vi "LabVIEW_MQTT_Toolkit_V2.vi"() -> ()   [LabVIEW 2021] (continued)
                n1873 = Close File(refnum=w4546, error in=w4544) -> (path=w4533:path)  [unwired: 1 out]
              }
              frame 16 {
                w4616 = T14 2 items=["User Home"=0, "User Desktop"=1, "User Documents"=2, "User Application Data"=3, "User Preferences"=4, "User Temporary"=5, "Public Documents"=6, "Public Application Data"=7, "Public Preferences"=8, "Public Cache"=13, "System Core Libraries"=9, "System Installed Libraries"=10, "Application Files"=11, "Boot Volume Root"=12] ("system directory type")
                n1874 = Decimate 1D Array(w4643) -> (w4641:dbl[])
                n1875 = Search and Replace String(replace all?=TRUE ("replace all? (F)"), input string=w4611, search string="/") -> (result string=w4632:string)  [unwired: 5 in, 3 out]
                n1876 = for {
                  tunnel: [w4665] -> w4640 mode=indexing
                  tunnel: w4642 -> [w4663] mode=indexing
                  tunnel: w4641 -> [w4662] mode=indexing
                  tunnel: [w4662] -> w4639 mode=indexing
                  tunnel: w4638 -> [w4657]
                  tunnel: w4637 -> [w4656]
                  tunnel: w4636 -> [w4655] mode=indexing
                  tunnel: w4635 -> [w4654]
                  tunnel: [w4648] -> w4634
                  n1877 = Join Numbers(hi=w4657, lo=w4656) -> ((hi.lo)=w4659:u32)
                  n1878 = To Double Precision Float(number=w4655) -> (double precision float=w4660:dbl)
                  n1879 = Number To Decimal String(number=w4663) -> (decimal integer string=w4664:string)  [unwired: 1 in]
                  n1880 = Number To Fractional String(number=w4662, precision (6)=i16 3 ("width (-)")) -> (F-format string=w4666:string)  [unwired: 2 in]
                  n1881 = Divide(x=w4660, y=w4654) -> (x/y=w4661:dbl)
                  n1882 = Build Array(w4664, w4666) -> (w4665:string[])
                  n1883 = To Unsigned Quad Integer(1:w4659) -> (0:w4658:u64)
                  n1884 = call "Unix Time to Timestamp.vi"("Fractional Second"=w4661, "Unix Time (s)"=w4658) -> ("Timestamp"=w4649:timestamp)  [unwired: 8 in, 1 out]
                  n1885 = Format Date/Time String(seconds (now)=w4649, UTC format=TRUE) -> (date/time string=w4650:string)  [unwired: 1 in]
                  n1886 = Scan From String(format string="%<%x %H:%M:%S%3u>T", input string=w4650) -> (output 1=w4651:timestamp)  [unwired: 3 in, 3 out]
                  n1887 = To Double Precision Float(number=w4651) -> (double precision float=w4648:dbl)
                }
                n1888 = Concatenate Strings(w4609, "TimeStamp;MeasureINC_Y(Deg)", "\n") -> (w4625:string)
                n1889 = Concatenate Strings(w4632, "_" ("string"), "S_E_T.csv") -> (w4633:string)
                n1890 = call <vilib>:"Get System Directory.vi"("system directory type"=w4616) -> ("system directory"=w4626:path)  [unwired: 10 in]
                n1891 = Build Path(base path=w4626, name or relative path="Logfile") -> (appended path=w4627:path)
                n1892 = call <vilib>:"Check if File or Folder Exists.vi"("path"=w4627) -> ("file or folder exists?"=w4628:bool, "dup path"=w4629:path)  [unwired: 8 in, 1 out]
                n1893 = case shown="False" w4628 {
                  tunnel: w4629 -> [w4646 w4647]
                  tunnel: [w4645 w4647] -> w4630
                  frame False {
                    n1894 = Create Folder(path (use dialog)=w4646) -> (created path=w4645:path)  [unwired: 2 in, 2 out]
                  }
                  frame True {
                  }
                }
                n1895 = Build Path(base path=w4630, name or relative path=w4633) -> (appended path=w4631:path)
                n1896 = Open/Create/Replace File(file path (use dialog)=w4631, operation (0:open)=T11."open or create") -> (refnum out=w4624:refnum<file>, error out=w4622:errorcluster)  [unwired: 4 in, 1 out]
                n1897 = Write to Text File(file (use dialog)=w4624, text=w4625, error in=w4622) -> (refnum out=w4623:refnum<file>, error out=w4621:errorcluster)  [unwired: 1 in, 1 out]
                n1898 = Close File(refnum=w4623, error in=w4621) -> (path=w4610:path)  [unwired: 1 out]
              }
              frame 17 {
                w4675 = T14 2 items=["User Home"=0, "User Desktop"=1, "User Documents"=2, "User Application Data"=3, "User Preferences"=4, "User Temporary"=5, "Public Documents"=6, "Public Application Data"=7, "Public Preferences"=8, "Public Cache"=13, "System Core Libraries"=9, "System Installed Libraries"=10, "Application Files"=11, "Boot Volume Root"=12] ("system directory type")
                n1899 = Decimate 1D Array(w4705) -> (w4701:dbl[], w4703:dbl[])
                n1900 = Search and Replace String(replace all?=TRUE ("replace all? (F)"), input string=w4670, search string="/") -> (result string=w4691:string)  [unwired: 5 in, 3 out]
                n1901 = for {
                  tunnel: [w4730] -> w4702 mode=indexing
                  tunnel: w4704 -> [w4728] mode=indexing
                  tunnel: w4701 -> [w4725] mode=indexing
                  tunnel: w4703 -> [w4724] mode=indexing
                  tunnel: [w4725] -> w4700 mode=indexing
                  tunnel: [w4724] -> w4699 mode=indexing
                  tunnel: w4698 -> [w4719]
                  tunnel: w4697 -> [w4718]
                  tunnel: w4696 -> [w4717] mode=indexing
                  tunnel: w4695 -> [w4716]
                  tunnel: [w4710] -> w4694
                  tunnel: [w4710] -> w4693
                  n1902 = Join Numbers(hi=w4719, lo=w4718) -> ((hi.lo)=w4721:u32)
                  n1903 = To Double Precision Float(number=w4717) -> (double precision float=w4722:dbl)
                  n1904 = Number To Decimal String(number=w4728) -> (decimal integer string=w4729:string)  [unwired: 1 in]
                  n1905 = Number To Fractional String(number=w4725, precision (6)=i16 3 ("width (-)")) -> (F-format string=w4731:string)  [unwired: 2 in]
                  n1906 = Number To Fractional String(number=w4724, precision (6)=i16 3 ("width (-)")) -> (F-format string=w4726:string)  [unwired: 2 in]
                  n1907 = Divide(x=w4722, y=w4716) -> (x/y=w4723:dbl)
                  n1908 = Build Array(w4729, w4731, w4726) -> (w4730:string[])
                  n1909 = To Unsigned Quad Integer(1:w4721) -> (0:w4720:u64)
                  n1910 = call "Unix Time to Timestamp.vi"("Fractional Second"=w4723, "Unix Time (s)"=w4720) -> ("Timestamp"=w4711:timestamp)  [unwired: 8 in, 1 out]
                  n1911 = Format Date/Time String(seconds (now)=w4711, UTC format=TRUE) -> (date/time string=w4712:string)  [unwired: 1 in]
                  n1912 = Scan From String(format string="%<%x %H:%M:%S%3u>T", input string=w4712) -> (output 1=w4713:timestamp)  [unwired: 3 in, 3 out]
                  n1913 = To Double Precision Float(number=w4713) -> (double precision float=w4710:dbl)
                }
                n1914 = Concatenate Strings(w4691, "_" ("string"), "S_E_T.csv") -> (w4692:string)
                n1915 = call <vilib>:"Get System Directory.vi"("system directory type"=w4675) -> ("system directory"=w4685:path)  [unwired: 10 in]
                n1916 = Concatenate Strings(w4668, "TimeStamp;MeasureCh_Z(g);INC_Y(Deg)", "\n") -> (w4684:string)
                n1917 = Build Path(base path=w4685, name or relative path="Logfile") -> (appended path=w4686:path)
                n1918 = call <vilib>:"Check if File or Folder Exists.vi"("path"=w4686) -> ("file or folder exists?"=w4687:bool, "dup path"=w4688:path)  [unwired: 8 in, 1 out]
                n1919 = case shown="False" w4687 {
                  tunnel: w4688 -> [w4708 w4709]
                  tunnel: [w4707 w4709] -> w4689
                  frame False {
                    n1920 = Create Folder(path (use dialog)=w4708) -> (created path=w4707:path)  [unwired: 2 in, 2 out]
                  }
                  frame True {
                  }
                }
                n1921 = Build Path(base path=w4689, name or relative path=w4692) -> (appended path=w4690:path)
                n1922 = Open/Create/Replace File(file path (use dialog)=w4690, operation (0:open)=T11."open or create") -> (refnum out=w4683:refnum<file>, error out=w4681:errorcluster)  [unwired: 4 in, 1 out]
                n1923 = Write to Text File(file (use dialog)=w4683, text=w4684, error in=w4681) -> (refnum out=w4682:refnum<file>, error out=w4680:errorcluster)  [unwired: 1 in, 1 out]
                n1924 = Close File(refnum=w4682, error in=w4680) -> (path=w4669:path)  [unwired: 1 out]
              }
              frame 18 {
                w4740 = T14 2 items=["User Home"=0, "User Desktop"=1, "User Documents"=2, "User Application Data"=3, "User Preferences"=4, "User Temporary"=5, "Public Documents"=6, "Public Application Data"=7, "Public Preferences"=8, "Public Cache"=13, "System Core Libraries"=9, "System Installed Libraries"=10, "Application Files"=11, "Boot Volume Root"=12] ("system directory type")
                n1925 = Decimate 1D Array(w4769) -> (w4765:dbl[], w4767:dbl[])
                n1926 = Search and Replace String(replace all?=TRUE ("replace all? (F)"), input string=w4734, search string="/") -> (result string=w4756:string)  [unwired: 5 in, 3 out]
                n1927 = Concatenate Strings(w4733, "TimeStamp;MeasureCh_X(g);INC_Y(Deg)", "\n") -> (w4749:string)
                n1928 = for {
                  tunnel: [w4794] -> w4766 mode=indexing
                  tunnel: w4768 -> [w4790] mode=indexing
                  tunnel: w4765 -> [w4789] mode=indexing
                  tunnel: w4767 -> [w4788] mode=indexing
                  tunnel: [w4789] -> w4764 mode=indexing
                  tunnel: [w4788] -> w4763 mode=indexing
                  tunnel: w4762 -> [w4783]
                  tunnel: w4761 -> [w4782]
                  tunnel: w4760 -> [w4781] mode=indexing
                  tunnel: w4759 -> [w4780]
                  tunnel: [w4774] -> w4758
                  n1929 = Join Numbers(hi=w4783, lo=w4782) -> ((hi.lo)=w4785:u32)
                  n1930 = To Double Precision Float(number=w4781) -> (double precision float=w4786:dbl)
                  n1931 = Number To Decimal String(number=w4790) -> (decimal integer string=w4793:string)  [unwired: 1 in]
                  n1932 = Number To Fractional String(number=w4789, precision (6)=i16 3 ("width (-)")) -> (F-format string=w4795:string)  [unwired: 2 in]
                  n1933 = Number To Fractional String(number=w4788, precision (6)=i16 3 ("width (-)")) -> (F-format string=w4791:string)  [unwired: 2 in]
                  n1934 = Divide(x=w4786, y=w4780) -> (x/y=w4787:dbl)
                  n1935 = Build Array(w4793, w4795, w4791) -> (w4794:string[])
                  n1936 = To Unsigned Quad Integer(1:w4785) -> (0:w4784:u64)
                  n1937 = call "Unix Time to Timestamp.vi"("Fractional Second"=w4787, "Unix Time (s)"=w4784) -> ("Timestamp"=w4775:timestamp)  [unwired: 8 in, 1 out]
                  n1938 = Format Date/Time String(seconds (now)=w4775, UTC format=TRUE) -> (date/time string=w4776:string)  [unwired: 1 in]
                  n1939 = Scan From String(format string="%<%x %H:%M:%S%3u>T", input string=w4776) -> (output 1=w4777:timestamp)  [unwired: 3 in, 3 out]
                  n1940 = To Double Precision Float(number=w4777) -> (double precision float=w4774:dbl)
                }
                n1941 = Concatenate Strings(w4756, "_" ("string"), "S_E_T.csv") -> (w4757:string)
                n1942 = call <vilib>:"Get System Directory.vi"("system directory type"=w4740) -> ("system directory"=w4750:path)  [unwired: 10 in]
                n1943 = Build Path(base path=w4750, name or relative path="Logfile") -> (appended path=w4751:path)
                n1944 = call <vilib>:"Check if File or Folder Exists.vi"("path"=w4751) -> ("file or folder exists?"=w4752:bool, "dup path"=w4753:path)  [unwired: 8 in, 1 out]
                n1945 = case shown="False" w4752 {
                  tunnel: w4753 -> [w4772 w4773]
                  tunnel: [w4771 w4773] -> w4754
                  frame False {
                    n1946 = Create Folder(path (use dialog)=w4772) -> (created path=w4771:path)  [unwired: 2 in, 2 out]
                  }
                  frame True {
                  }
                }
                n1947 = Build Path(base path=w4754, name or relative path=w4757) -> (appended path=w4755:path)
                n1948 = Open/Create/Replace File(file path (use dialog)=w4755, operation (0:open)=T11."open or create") -> (refnum out=w4748:refnum<file>, error out=w4746:errorcluster)  [unwired: 4 in, 1 out]
                n1949 = Write to Text File(file (use dialog)=w4748, text=w4749, error in=w4746) -> (refnum out=w4747:refnum<file>, error out=w4745:errorcluster)  [unwired: 1 in, 1 out]
                n1950 = Close File(refnum=w4747, error in=w4745) -> (path=w4735:path)  [unwired: 1 out]
              }
              frame 19 {
                w4804 = T14 2 items=["User Home"=0, "User Desktop"=1, "User Documents"=2, "User Application Data"=3, "User Preferences"=4, "User Temporary"=5, "Public Documents"=6, "Public Application Data"=7, "Public Preferences"=8, "Public Cache"=13, "System Core Libraries"=9, "System Installed Libraries"=10, "Application Files"=11, "Boot Volume Root"=12] ("system directory type")
                n1951 = Search and Replace String(replace all?=TRUE ("replace all? (F)"), input string=w4799, search string="/") -> (result string=w4820:string)  [unwired: 5 in, 3 out]
                n1952 = Concatenate Strings(w4820, "_" ("string"), "S_E_T.csv") -> (w4821:string)
                n1953 = call <vilib>:"Get System Directory.vi"("system directory type"=w4804) -> ("system directory"=w4814:path)  [unwired: 10 in]
                n1954 = Concatenate Strings(w4797, "TimeStamp;MeasureCh_Z(g);Ch_X(g);INC_Y(Deg)", "\n") -> (w4813:string)
                n1955 = Decimate 1D Array(w4837) -> (w4833:dbl[], w4832:dbl[], w4835:dbl[])
                n1956 = for {
                  tunnel: [w4865] -> w4834 mode=indexing
                  tunnel: w4836 -> [w4859] mode=indexing
                  tunnel: w4833 -> [w4858] mode=indexing
                  tunnel: w4832 -> [w4857] mode=indexing
                  tunnel: w4835 -> [w4856] mode=indexing
                  tunnel: [w4858] -> w4831 mode=indexing
                  tunnel: [w4857] -> w4830 mode=indexing
                  tunnel: [w4856] -> w4829 mode=indexing
                  tunnel: w4828 -> [w4851]
                  tunnel: w4827 -> [w4850]
                  tunnel: w4826 -> [w4849] mode=indexing
                  tunnel: w4825 -> [w4848]
                  tunnel: [w4842] -> w4824
                  tunnel: [w4842] -> w4823
                  tunnel: [w4842] -> w4822
                  n1957 = Join Numbers(hi=w4851, lo=w4850) -> ((hi.lo)=w4853:u32)
                  n1958 = To Double Precision Float(number=w4849) -> (double precision float=w4854:dbl)
                  n1959 = Number To Decimal String(number=w4859) -> (decimal integer string=w4864:string)  [unwired: 1 in]
                  n1960 = Number To Fractional String(number=w4858, precision (6)=i16 3 ("width (-)")) -> (F-format string=w4866:string)  [unwired: 2 in]
                  n1961 = Number To Fractional String(number=w4857, precision (6)=i16 3 ("width (-)")) -> (F-format string=w4862:string)  [unwired: 2 in]
                  n1962 = Number To Fractional String(number=w4856, precision (6)=i16 3 ("width (-)")) -> (F-format string=w4860:string)  [unwired: 2 in]
                  n1963 = Build Array(w4864, w4866, w4862, w4860) -> (w4865:string[])
                  n1964 = Divide(x=w4854, y=w4848) -> (x/y=w4855:dbl)
                  n1965 = To Unsigned Quad Integer(1:w4853) -> (0:w4852:u64)
                  n1966 = call "Unix Time to Timestamp.vi"("Fractional Second"=w4855, "Unix Time (s)"=w4852) -> ("Timestamp"=w4843:timestamp)  [unwired: 8 in, 1 out]
                  n1967 = Format Date/Time String(seconds (now)=w4843, UTC format=TRUE) -> (date/time string=w4844:string)  [unwired: 1 in]
                  n1968 = Scan From String(format string="%<%x %H:%M:%S%3u>T", input string=w4844) -> (output 1=w4845:timestamp)  [unwired: 3 in, 3 out]
                  n1969 = To Double Precision Float(number=w4845) -> (double precision float=w4842:dbl)
                }
                n1970 = Build Path(base path=w4814, name or relative path="Logfile") -> (appended path=w4815:path)
                n1971 = call <vilib>:"Check if File or Folder Exists.vi"("path"=w4815) -> ("file or folder exists?"=w4816:bool, "dup path"=w4817:path)  [unwired: 8 in, 1 out]
                n1972 = case shown="False" w4816 {
                  tunnel: w4817 -> [w4840 w4841]
                  tunnel: [w4839 w4841] -> w4818
                  frame False {
                    n1973 = Create Folder(path (use dialog)=w4840) -> (created path=w4839:path)  [unwired: 2 in, 2 out]
                  }
                  frame True {
                  }
                }
                n1974 = Build Path(base path=w4818, name or relative path=w4821) -> (appended path=w4819:path)
                n1975 = Open/Create/Replace File(file path (use dialog)=w4819, operation (0:open)=T11."open or create") -> (refnum out=w4812:refnum<file>, error out=w4810:errorcluster)  [unwired: 4 in, 1 out]
                n1976 = Write to Text File(file (use dialog)=w4812, text=w4813, error in=w4810) -> (refnum out=w4811:refnum<file>, error out=w4809:errorcluster)  [unwired: 1 in, 1 out]
                n1977 = Close File(refnum=w4811, error in=w4809) -> (path=w4798:path)  [unwired: 1 out]
              }
              frame 20 {
                w4875 = T14 2 items=["User Home"=0, "User Desktop"=1, "User Documents"=2, "User Application Data"=3, "User Preferences"=4, "User Temporary"=5, "Public Documents"=6, "Public Application Data"=7, "Public Preferences"=8, "Public Cache"=13, "System Core Libraries"=9, "System Installed Libraries"=10, "Application Files"=11, "Boot Volume Root"=12] ("system directory type")
                n1978 = Decimate 1D Array(w4904) -> (w4900:dbl[], w4902:dbl[])
                n1979 = Search and Replace String(replace all?=TRUE ("replace all? (F)"), input string=w4869, search string="/") -> (result string=w4891:string)  [unwired: 5 in, 3 out]
                n1980 = for {
                  tunnel: [w4929] -> w4901 mode=indexing
                  tunnel: w4903 -> [w4925] mode=indexing
                  tunnel: w4900 -> [w4924] mode=indexing
                  tunnel: w4902 -> [w4923] mode=indexing
                  tunnel: [w4924] -> w4899 mode=indexing
                  tunnel: [w4923] -> w4898 mode=indexing
                  tunnel: w4897 -> [w4918]
                  tunnel: w4896 -> [w4917]
                  tunnel: w4895 -> [w4916] mode=indexing
                  tunnel: w4894 -> [w4915]
                  tunnel: [w4909] -> w4893
                  n1981 = Join Numbers(hi=w4918, lo=w4917) -> ((hi.lo)=w4920:u32)
                  n1982 = To Double Precision Float(number=w4916) -> (double precision float=w4921:dbl)
                  n1983 = Number To Decimal String(number=w4925) -> (decimal integer string=w4928:string)  [unwired: 1 in]
                  n1984 = Number To Fractional String(number=w4924, precision (6)=i16 3 ("width (-)")) -> (F-format string=w4930:string)  [unwired: 2 in]
                  n1985 = Number To Fractional String(number=w4923, precision (6)=i16 3 ("width (-)")) -> (F-format string=w4926:string)  [unwired: 2 in]
                  n1986 = Divide(x=w4921, y=w4915) -> (x/y=w4922:dbl)
                  n1987 = Build Array(w4928, w4930, w4926) -> (w4929:string[])
                  n1988 = To Unsigned Quad Integer(1:w4920) -> (0:w4919:u64)
                  n1989 = call "Unix Time to Timestamp.vi"("Fractional Second"=w4922, "Unix Time (s)"=w4919) -> ("Timestamp"=w4910:timestamp)  [unwired: 8 in, 1 out]
                  n1990 = Format Date/Time String(seconds (now)=w4910, UTC format=TRUE) -> (date/time string=w4911:string)  [unwired: 1 in]
                  n1991 = Scan From String(format string="%<%x %H:%M:%S%3u>T", input string=w4911) -> (output 1=w4912:timestamp)  [unwired: 3 in, 3 out]
                  n1992 = To Double Precision Float(number=w4912) -> (double precision float=w4909:dbl)
                }
                n1993 = Concatenate Strings(w4868, "TimeStamp;MeasureCh_Y(g);INC_Y(Deg)", "\n") -> (w4884:string)
                n1994 = Concatenate Strings(w4891, "_" ("string"), "S_E_T.csv") -> (w4892:string)
                n1995 = call <vilib>:"Get System Directory.vi"("system directory type"=w4875) -> ("system directory"=w4885:path)  [unwired: 10 in]
                n1996 = Build Path(base path=w4885, name or relative path="Logfile") -> (appended path=w4886:path)
                n1997 = call <vilib>:"Check if File or Folder Exists.vi"("path"=w4886) -> ("file or folder exists?"=w4887:bool, "dup path"=w4888:path)  [unwired: 8 in, 1 out]
                n1998 = case shown="False" w4887 {
                  tunnel: w4888 -> [w4907 w4908]
                  tunnel: [w4906 w4908] -> w4889
                  frame False {
                    n1999 = Create Folder(path (use dialog)=w4907) -> (created path=w4906:path)  [unwired: 2 in, 2 out]
                  }
                  frame True {
                  }
                }
                n2000 = Build Path(base path=w4889, name or relative path=w4892) -> (appended path=w4890:path)
                n2001 = Open/Create/Replace File(file path (use dialog)=w4890, operation (0:open)=T11."open or create") -> (refnum out=w4883:refnum<file>, error out=w4881:errorcluster)  [unwired: 4 in, 1 out]
                n2002 = Write to Text File(file (use dialog)=w4883, text=w4884, error in=w4881) -> (refnum out=w4882:refnum<file>, error out=w4880:errorcluster)  [unwired: 1 in, 1 out]
                n2003 = Close File(refnum=w4882, error in=w4880) -> (path=w4870:path)  [unwired: 1 out]
              }
              frame 21 {
                w4939 = T14 2 items=["User Home"=0, "User Desktop"=1, "User Documents"=2, "User Application Data"=3, "User Preferences"=4, "User Temporary"=5, "Public Documents"=6, "Public Application Data"=7, "Public Preferences"=8, "Public Cache"=13, "System Core Libraries"=9, "System Installed Libraries"=10, "Application Files"=11, "Boot Volume Root"=12] ("system directory type")
                n2004 = Search and Replace String(replace all?=TRUE ("replace all? (F)"), input string=w4934, search string="/") -> (result string=w4955:string)  [unwired: 5 in, 3 out]
                n2005 = Concatenate Strings(w4932, "TimeStamp;MeasureCh_Z(g);Ch_Y(g);INC_Y(Deg)", "\n") -> (w4948:string)
                n2006 = Concatenate Strings(w4955, "_" ("string"), "S_E_T.csv") -> (w4956:string)
                n2007 = call <vilib>:"Get System Directory.vi"("system directory type"=w4939) -> ("system directory"=w4949:path)  [unwired: 10 in]
                n2008 = Decimate 1D Array(w4972) -> (w4968:dbl[], w4967:dbl[], w4970:dbl[])
                n2009 = for {
                  tunnel: [w5000] -> w4969 mode=indexing
                  tunnel: w4971 -> [w4994] mode=indexing
                  tunnel: w4968 -> [w4993] mode=indexing
                  tunnel: w4967 -> [w4992] mode=indexing
                  tunnel: w4970 -> [w4991] mode=indexing
                  tunnel: [w4993] -> w4966 mode=indexing
                  tunnel: [w4992] -> w4965 mode=indexing
                  tunnel: [w4991] -> w4964 mode=indexing
                  tunnel: w4963 -> [w4986]
                  tunnel: w4962 -> [w4985]
                  tunnel: w4961 -> [w4984] mode=indexing
                  tunnel: w4960 -> [w4983]
                  tunnel: [w4977] -> w4959
                  tunnel: [w4977] -> w4958
                  tunnel: [w4977] -> w4957
                  n2010 = Join Numbers(hi=w4986, lo=w4985) -> ((hi.lo)=w4988:u32)
                  n2011 = To Double Precision Float(number=w4984) -> (double precision float=w4989:dbl)
                  n2012 = Number To Decimal String(number=w4994) -> (decimal integer string=w4999:string)  [unwired: 1 in]
                  n2013 = Number To Fractional String(number=w4993, precision (6)=i16 3 ("width (-)")) -> (F-format string=w5001:string)  [unwired: 2 in]
                  n2014 = Number To Fractional String(number=w4992, precision (6)=i16 3 ("width (-)")) -> (F-format string=w4997:string)  [unwired: 2 in]
                  n2015 = Number To Fractional String(number=w4991, precision (6)=i16 3 ("width (-)")) -> (F-format string=w4995:string)  [unwired: 2 in]
                  n2016 = Build Array(w4999, w5001, w4997, w4995) -> (w5000:string[])
                  n2017 = Divide(x=w4989, y=w4983) -> (x/y=w4990:dbl)
                  n2018 = To Unsigned Quad Integer(1:w4988) -> (0:w4987:u64)
                  n2019 = call "Unix Time to Timestamp.vi"("Fractional Second"=w4990, "Unix Time (s)"=w4987) -> ("Timestamp"=w4978:timestamp)  [unwired: 8 in, 1 out]
                  n2020 = Format Date/Time String(seconds (now)=w4978, UTC format=TRUE) -> (date/time string=w4979:string)  [unwired: 1 in]
                  n2021 = Scan From String(format string="%<%x %H:%M:%S%3u>T", input string=w4979) -> (output 1=w4980:timestamp)  [unwired: 3 in, 3 out]
                  n2022 = To Double Precision Float(number=w4980) -> (double precision float=w4977:dbl)
                }
                n2023 = Build Path(base path=w4949, name or relative path="Logfile") -> (appended path=w4950:path)
                n2024 = call <vilib>:"Check if File or Folder Exists.vi"("path"=w4950) -> ("file or folder exists?"=w4951:bool, "dup path"=w4952:path)  [unwired: 8 in, 1 out]
                n2025 = case shown="False" w4951 {
                  tunnel: w4952 -> [w4975 w4976]
                  tunnel: [w4974 w4976] -> w4953
                  frame False {
                    n2026 = Create Folder(path (use dialog)=w4975) -> (created path=w4974:path)  [unwired: 2 in, 2 out]
                  }
                  frame True {
                  }
                }
                n2027 = Build Path(base path=w4953, name or relative path=w4956) -> (appended path=w4954:path)
                n2028 = Open/Create/Replace File(file path (use dialog)=w4954, operation (0:open)=T11."open or create") -> (refnum out=w4947:refnum<file>, error out=w4945:errorcluster)  [unwired: 4 in, 1 out]
                n2029 = Write to Text File(file (use dialog)=w4947, text=w4948, error in=w4945) -> (refnum out=w4946:refnum<file>, error out=w4944:errorcluster)  [unwired: 1 in, 1 out]
                n2030 = Close File(refnum=w4946, error in=w4944) -> (path=w4933:path)  [unwired: 1 out]
              }
              frame 22 {
                w5010 = T14 2 items=["User Home"=0, "User Desktop"=1, "User Documents"=2, "User Application Data"=3, "User Preferences"=4, "User Temporary"=5, "Public Documents"=6, "Public Application Data"=7, "Public Preferences"=8, "Public Cache"=13, "System Core Libraries"=9, "System Installed Libraries"=10, "Application Files"=11, "Boot Volume Root"=12] ("system directory type")
                n2031 = Search and Replace String(replace all?=TRUE ("replace all? (F)"), input string=w5005, search string="/") -> (result string=w5026:string)  [unwired: 5 in, 3 out]
                n2032 = Concatenate Strings(w5003, "TimeStamp;MeasureCh_X(g);Ch_Y(g);INC_X(Deg)", "\n") -> (w5019:string)
                n2033 = Concatenate Strings(w5026, "_" ("string"), "S_E_T.csv") -> (w5027:string)
                n2034 = call <vilib>:"Get System Directory.vi"("system directory type"=w5010) -> ("system directory"=w5020:path)  [unwired: 10 in]
                n2035 = Decimate 1D Array(w5043) -> (w5039:dbl[], w5038:dbl[], w5042:dbl[])
                n2036 = for {
                  tunnel: [w5071] -> w5040 mode=indexing
                  tunnel: w5041 -> [w5065] mode=indexing
                  tunnel: w5039 -> [w5064] mode=indexing
                  tunnel: w5038 -> [w5063] mode=indexing
                  tunnel: w5042 -> [w5062] mode=indexing
                  tunnel: [w5064] -> w5037 mode=indexing
                  tunnel: [w5063] -> w5036 mode=indexing
                  tunnel: [w5062] -> w5035 mode=indexing
                  tunnel: w5034 -> [w5057]
                  tunnel: w5033 -> [w5056]
                  tunnel: w5032 -> [w5055] mode=indexing
                  tunnel: w5031 -> [w5054]
                  tunnel: [w5048] -> w5030
                  tunnel: [w5048] -> w5029
                  tunnel: [w5048] -> w5028
                  n2037 = Join Numbers(hi=w5057, lo=w5056) -> ((hi.lo)=w5059:u32)
                  n2038 = To Double Precision Float(number=w5055) -> (double precision float=w5060:dbl)
                  n2039 = Number To Decimal String(number=w5065) -> (decimal integer string=w5070:string)  [unwired: 1 in]
                  n2040 = Number To Fractional String(number=w5064, precision (6)=i16 3 ("width (-)")) -> (F-format string=w5072:string)  [unwired: 2 in]
                  n2041 = Number To Fractional String(number=w5063, precision (6)=i16 3 ("width (-)")) -> (F-format string=w5068:string)  [unwired: 2 in]
                  n2042 = Number To Fractional String(number=w5062, precision (6)=i16 3 ("width (-)")) -> (F-format string=w5066:string)  [unwired: 2 in]
                  n2043 = Build Array(w5070, w5072, w5068, w5066) -> (w5071:string[])
                  n2044 = Divide(x=w5060, y=w5054) -> (x/y=w5061:dbl)
                  n2045 = To Unsigned Quad Integer(1:w5059) -> (0:w5058:u64)
                  n2046 = call "Unix Time to Timestamp.vi"("Fractional Second"=w5061, "Unix Time (s)"=w5058) -> ("Timestamp"=w5049:timestamp)  [unwired: 8 in, 1 out]
                  n2047 = Format Date/Time String(seconds (now)=w5049, UTC format=TRUE) -> (date/time string=w5050:string)  [unwired: 1 in]
                  n2048 = Scan From String(format string="%<%x %H:%M:%S%3u>T", input string=w5050) -> (output 1=w5051:timestamp)  [unwired: 3 in, 3 out]
                  n2049 = To Double Precision Float(number=w5051) -> (double precision float=w5048:dbl)
                }
                n2050 = Build Path(base path=w5020, name or relative path="Logfile") -> (appended path=w5021:path)
                n2051 = call <vilib>:"Check if File or Folder Exists.vi"("path"=w5021) -> ("file or folder exists?"=w5022:bool, "dup path"=w5023:path)  [unwired: 8 in, 1 out]
                n2052 = case shown="False" w5022 {
                  tunnel: w5023 -> [w5046 w5047]
                  tunnel: [w5045 w5047] -> w5024
                  frame False {
                    n2053 = Create Folder(path (use dialog)=w5046) -> (created path=w5045:path)  [unwired: 2 in, 2 out]
                  }
                  frame True {
                  }
                }
                n2054 = Build Path(base path=w5024, name or relative path=w5027) -> (appended path=w5025:path)
                n2055 = Open/Create/Replace File(file path (use dialog)=w5025, operation (0:open)=T11."open or create") -> (refnum out=w5018:refnum<file>, error out=w5016:errorcluster)  [unwired: 4 in, 1 out]
                n2056 = Write to Text File(file (use dialog)=w5018, text=w5019, error in=w5016) -> (refnum out=w5017:refnum<file>, error out=w5015:errorcluster)  [unwired: 1 in, 1 out]
                n2057 = Close File(refnum=w5017, error in=w5015) -> (path=w5004:path)  [unwired: 1 out]
              }
              frame 23 {
                w5081 = T14 2 items=["User Home"=0, "User Desktop"=1, "User Documents"=2, "User Application Data"=3, "User Preferences"=4, "User Temporary"=5, "Public Documents"=6, "Public Application Data"=7, "Public Preferences"=8, "Public Cache"=13, "System Core Libraries"=9, "System Installed Libraries"=10, "Application Files"=11, "Boot Volume Root"=12] ("system directory type")
                n2058 = Search and Replace String(replace all?=TRUE ("replace all? (F)"), input string=w5075, search string="/") -> (result string=w5097:string)  [unwired: 5 in, 3 out]
                n2059 = Concatenate Strings(w5074, "TimeStamp;MeasureCh_Z(g);Ch_X(g);Ch_Y(g);INC_Y(Deg)", "\n") -> (w5090:string)
                n2060 = Concatenate Strings(w5097, "_" ("string"), "S_E_T.csv") -> (w5098:string)
                n2061 = call <vilib>:"Get System Directory.vi"("system directory type"=w5081) -> ("system directory"=w5091:path)  [unwired: 10 in]
                n2062 = Decimate 1D Array(w5114) -> (w5113:dbl[], w5112:dbl[], w5111:dbl[], w5108:dbl[])
                n2063 = for {
                  tunnel: [w5144] -> w5109 mode=indexing
                  tunnel: w5110 -> [w5138] mode=indexing
                  tunnel: w5113 -> [w5136] mode=indexing
                  tunnel: w5112 -> [w5135] mode=indexing
                  tunnel: w5111 -> [w5134] mode=indexing
                  tunnel: w5108 -> [w5133] mode=indexing
                  tunnel: [w5136] -> w5107 mode=indexing
                  tunnel: [w5135] -> w5106 mode=indexing
                  tunnel: [w5134] -> w5105 mode=indexing
                  tunnel: [w5133] -> w5104 mode=indexing
                  tunnel: w5103 -> [w5128]
                  tunnel: w5102 -> [w5127]
                  tunnel: w5101 -> [w5126] mode=indexing
                  tunnel: w5100 -> [w5125]
                  tunnel: [w5119] -> w5099
                  n2064 = Number To Fractional String(number=w5133, precision (6)=i16 3 ("width (-)")) -> ()  [unwired: 2 in, 1 out]
                  n2065 = Join Numbers(hi=w5128, lo=w5127) -> ((hi.lo)=w5130:u32)
                  n2066 = To Double Precision Float(number=w5126) -> (double precision float=w5131:dbl)
                  n2067 = Number To Decimal String(number=w5138) -> (decimal integer string=w5143:string)  [unwired: 1 in]
                  n2068 = Number To Fractional String(number=w5136, precision (6)=i16 3 ("width (-)")) -> (F-format string=w5145:string)  [unwired: 2 in]
                  n2069 = Number To Fractional String(number=w5135, precision (6)=i16 3 ("width (-)")) -> (F-format string=w5141:string)  [unwired: 2 in]
                  n2070 = Number To Fractional String(number=w5134, precision (6)=i16 3 ("width (-)")) -> (F-format string=w5139:string)  [unwired: 2 in]
                  n2071 = Build Array(w5143, w5145, w5141, w5139) -> (w5144:string[])
                  n2072 = Divide(x=w5131, y=w5125) -> (x/y=w5132:dbl)
                  n2073 = To Unsigned Quad Integer(1:w5130) -> (0:w5129:u64)
                  n2074 = call "Unix Time to Timestamp.vi"("Fractional Second"=w5132, "Unix Time (s)"=w5129) -> ("Timestamp"=w5120:timestamp)  [unwired: 8 in, 1 out]
                  n2075 = Format Date/Time String(seconds (now)=w5120, UTC format=TRUE) -> (date/time string=w5121:string)  [unwired: 1 in]
                  n2076 = Scan From String(format string="%<%x %H:%M:%S%3u>T", input string=w5121) -> (output 1=w5122:timestamp)  [unwired: 3 in, 3 out]
                  n2077 = To Double Precision Float(number=w5122) -> (double precision float=w5119:dbl)
                }
                n2078 = Build Path(base path=w5091, name or relative path="Logfile") -> (appended path=w5092:path)
                n2079 = call <vilib>:"Check if File or Folder Exists.vi"("path"=w5092) -> ("file or folder exists?"=w5093:bool, "dup path"=w5094:path)  [unwired: 8 in, 1 out]
                n2080 = case shown="False" w5093 {
                  tunnel: w5094 -> [w5117 w5118]
                  tunnel: [w5116 w5118] -> w5095
                  frame False {
                    n2081 = Create Folder(path (use dialog)=w5117) -> (created path=w5116:path)  [unwired: 2 in, 2 out]
                  }
                  frame True {
                  }
                }
                n2082 = Build Path(base path=w5095, name or relative path=w5098) -> (appended path=w5096:path)
                n2083 = Open/Create/Replace File(file path (use dialog)=w5096, operation (0:open)=T11."open or create") -> (refnum out=w5089:refnum<file>, error out=w5087:errorcluster)  [unwired: 4 in, 1 out]
                n2084 = Write to Text File(file (use dialog)=w5089, text=w5090, error in=w5087) -> (refnum out=w5088:refnum<file>, error out=w5086:errorcluster)  [unwired: 1 in, 1 out]
                n2085 = Close File(refnum=w5088, error in=w5086) -> (path=w5076:path)  [unwired: 1 out]
              }
              frame 24 {
                w5154 = T14 2 items=["User Home"=0, "User Desktop"=1, "User Documents"=2, "User Application Data"=3, "User Preferences"=4, "User Temporary"=5, "Public Documents"=6, "Public Application Data"=7, "Public Preferences"=8, "Public Cache"=13, "System Core Libraries"=9, "System Installed Libraries"=10, "Application Files"=11, "Boot Volume Root"=12] ("system directory type")
                n2086 = Decimate 1D Array(w5183) -> (w5181:dbl[], w5180:dbl[])
                n2087 = Search and Replace String(replace all?=TRUE ("replace all? (F)"), input string=w5149, search string="/") -> (result string=w5170:string)  [unwired: 5 in, 3 out]
                n2088 = Concatenate Strings(w5147, "TimeStamp;Measure INC_X(Deg);INC_Y(Deg)", "\n") -> (w5163:string)
                n2089 = for {
                  tunnel: [w5208] -> w5179 mode=indexing
                  tunnel: w5182 -> [w5204] mode=indexing
                  tunnel: w5181 -> [w5203] mode=indexing
                  tunnel: w5180 -> [w5202] mode=indexing
                  tunnel: [w5203] -> w5178 mode=indexing
                  tunnel: [w5202] -> w5177 mode=indexing
                  tunnel: w5176 -> [w5197]
                  tunnel: w5175 -> [w5196]
                  tunnel: w5174 -> [w5195] mode=indexing
                  tunnel: w5173 -> [w5194]
                  tunnel: [w5188] -> w5172
                  n2090 = Join Numbers(hi=w5197, lo=w5196) -> ((hi.lo)=w5199:u32)
                  n2091 = To Double Precision Float(number=w5195) -> (double precision float=w5200:dbl)
                  n2092 = Number To Decimal String(number=w5204) -> (decimal integer string=w5207:string)  [unwired: 1 in]
                  n2093 = Number To Fractional String(number=w5203, precision (6)=i16 3 ("width (-)")) -> (F-format string=w5209:string)  [unwired: 2 in]
                  n2094 = Number To Fractional String(number=w5202, precision (6)=i16 3 ("width (-)")) -> (F-format string=w5205:string)  [unwired: 2 in]
                  n2095 = Divide(x=w5200, y=w5194) -> (x/y=w5201:dbl)
                  n2096 = Build Array(w5207, w5209, w5205) -> (w5208:string[])
                  n2097 = To Unsigned Quad Integer(1:w5199) -> (0:w5198:u64)
                  n2098 = call "Unix Time to Timestamp.vi"("Fractional Second"=w5201, "Unix Time (s)"=w5198) -> ("Timestamp"=w5189:timestamp)  [unwired: 8 in, 1 out]
                  n2099 = Format Date/Time String(seconds (now)=w5189, UTC format=TRUE) -> (date/time string=w5190:string)  [unwired: 1 in]
                  n2100 = Scan From String(format string="%<%x %H:%M:%S%3u>T", input string=w5190) -> (output 1=w5191:timestamp)  [unwired: 3 in, 3 out]
                  n2101 = To Double Precision Float(number=w5191) -> (double precision float=w5188:dbl)
                }
                n2102 = Concatenate Strings(w5170, "_" ("string"), "S_E_T.csv") -> (w5171:string)
                n2103 = call <vilib>:"Get System Directory.vi"("system directory type"=w5154) -> ("system directory"=w5164:path)  [unwired: 10 in]
                n2104 = Build Path(base path=w5164, name or relative path="Logfile") -> (appended path=w5165:path)
                n2105 = call <vilib>:"Check if File or Folder Exists.vi"("path"=w5165) -> ("file or folder exists?"=w5166:bool, "dup path"=w5167:path)  [unwired: 8 in, 1 out]
                n2106 = case shown="False" w5166 {
                  tunnel: w5167 -> [w5186 w5187]
                  tunnel: [w5185 w5187] -> w5168
                  frame False {
                    n2107 = Create Folder(path (use dialog)=w5186) -> (created path=w5185:path)  [unwired: 2 in, 2 out]
                  }
                  frame True {
                  }
                }
                n2108 = Build Path(base path=w5168, name or relative path=w5171) -> (appended path=w5169:path)
                n2109 = Open/Create/Replace File(file path (use dialog)=w5169, operation (0:open)=T11."open or create") -> (refnum out=w5162:refnum<file>, error out=w5160:errorcluster)  [unwired: 4 in, 1 out]
                n2110 = Write to Text File(file (use dialog)=w5162, text=w5163, error in=w5160) -> (refnum out=w5161:refnum<file>, error out=w5159:errorcluster)  [unwired: 1 in, 1 out]
                n2111 = Close File(refnum=w5161, error in=w5159) -> (path=w5148:path)  [unwired: 1 out]
              }
              frame 25 {
                w5218 = T14 2 items=["User Home"=0, "User Desktop"=1, "User Documents"=2, "User Application Data"=3, "User Preferences"=4, "User Temporary"=5, "Public Documents"=6, "Public Application Data"=7, "Public Preferences"=8, "Public Cache"=13, "System Core Libraries"=9, "System Installed Libraries"=10, "Application Files"=11, "Boot Volume Root"=12] ("system directory type")
                n2112 = Search and Replace String(replace all?=TRUE ("replace all? (F)"), input string=w5213, search string="/") -> (result string=w5234:string)  [unwired: 5 in, 3 out]
                n2113 = Concatenate Strings(w5211, "TimeStamp;Measure Ch_Z(g);INC_X(Deg);INC_Y(Deg)", "\n") -> (w5227:string)
                n2114 = Concatenate Strings(w5234, "_" ("string"), "S_E_T.csv") -> (w5235:string)
                n2115 = call <vilib>:"Get System Directory.vi"("system directory type"=w5218) -> ("system directory"=w5228:path)  [unwired: 10 in]
                n2116 = Decimate 1D Array(w5249) -> (w5244:dbl[], w5247:dbl[], w5246:dbl[])
                n2117 = for {
                  tunnel: [w5277] -> w5245 mode=indexing
                  tunnel: w5248 -> [w5271] mode=indexing
                  tunnel: w5244 -> [w5270] mode=indexing
                  tunnel: w5247 -> [w5269] mode=indexing
                  tunnel: w5246 -> [w5268] mode=indexing
                  tunnel: [w5270] -> w5243 mode=indexing
                  tunnel: [w5269] -> w5242 mode=indexing
                  tunnel: [w5268] -> w5241 mode=indexing
                  tunnel: w5240 -> [w5263]
                  tunnel: w5239 -> [w5262]
                  tunnel: w5238 -> [w5261] mode=indexing
                  tunnel: w5237 -> [w5260]
                  tunnel: [w5254] -> w5236
                  n2118 = Join Numbers(hi=w5263, lo=w5262) -> ((hi.lo)=w5265:u32)
                  n2119 = To Double Precision Float(number=w5261) -> (double precision float=w5266:dbl)
                  n2120 = Number To Decimal String(number=w5271) -> (decimal integer string=w5276:string)  [unwired: 1 in]
                  n2121 = Number To Fractional String(number=w5270, precision (6)=i16 3 ("width (-)")) -> (F-format string=w5278:string)  [unwired: 2 in]
                  n2122 = Number To Fractional String(number=w5269, precision (6)=i16 3 ("width (-)")) -> (F-format string=w5274:string)  [unwired: 2 in]
                  n2123 = Number To Fractional String(number=w5268, precision (6)=i16 3 ("width (-)")) -> (F-format string=w5272:string)  [unwired: 2 in]
                  n2124 = Build Array(w5276, w5278, w5274, w5272) -> (w5277:string[])
                  n2125 = Divide(x=w5266, y=w5260) -> (x/y=w5267:dbl)
                  n2126 = To Unsigned Quad Integer(1:w5265) -> (0:w5264:u64)
                  n2127 = call "Unix Time to Timestamp.vi"("Fractional Second"=w5267, "Unix Time (s)"=w5264) -> ("Timestamp"=w5255:timestamp)  [unwired: 8 in, 1 out]
                  n2128 = Format Date/Time String(seconds (now)=w5255, UTC format=TRUE) -> (date/time string=w5256:string)  [unwired: 1 in]
                  n2129 = Scan From String(format string="%<%x %H:%M:%S%3u>T", input string=w5256) -> (output 1=w5257:timestamp)  [unwired: 3 in, 3 out]
                  n2130 = To Double Precision Float(number=w5257) -> (double precision float=w5254:dbl)
                }
                n2131 = Build Path(base path=w5228, name or relative path="Logfile") -> (appended path=w5229:path)
                n2132 = call <vilib>:"Check if File or Folder Exists.vi"("path"=w5229) -> ("file or folder exists?"=w5230:bool, "dup path"=w5231:path)  [unwired: 8 in, 1 out]
                n2133 = case shown="False" w5230 {
                  tunnel: w5231 -> [w5252 w5253]
                  tunnel: [w5251 w5253] -> w5232
                  frame False {
                    n2134 = Create Folder(path (use dialog)=w5252) -> (created path=w5251:path)  [unwired: 2 in, 2 out]
                  }
                  frame True {
                  }
                }
                n2135 = Build Path(base path=w5232, name or relative path=w5235) -> (appended path=w5233:path)
                n2136 = Open/Create/Replace File(file path (use dialog)=w5233, operation (0:open)=T11."open or create") -> (refnum out=w5226:refnum<file>, error out=w5224:errorcluster)  [unwired: 4 in, 1 out]
                n2137 = Write to Text File(file (use dialog)=w5226, text=w5227, error in=w5224) -> (refnum out=w5225:refnum<file>, error out=w5223:errorcluster)  [unwired: 1 in, 1 out]
                n2138 = Close File(refnum=w5225, error in=w5223) -> (path=w5212:path)  [unwired: 1 out]
              }
              frame 26 {
                w5287 = T14 2 items=["User Home"=0, "User Desktop"=1, "User Documents"=2, "User Application Data"=3, "User Preferences"=4, "User Temporary"=5, "Public Documents"=6, "Public Application Data"=7, "Public Preferences"=8, "Public Cache"=13, "System Core Libraries"=9, "System Installed Libraries"=10, "Application Files"=11, "Boot Volume Root"=12] ("system directory type")
                n2139 = Search and Replace String(replace all?=TRUE ("replace all? (F)"), input string=w5282, search string="/") -> (result string=w5303:string)  [unwired: 5 in, 3 out]
                n2140 = Concatenate Strings(w5280, "TimeStamp;Measure Ch_X(g);INC_X(Deg);INC_Y(Deg)", "\n") -> (w5296:string)
                n2141 = Concatenate Strings(w5303, "_" ("string"), "S_E_T.csv") -> (w5304:string)
                n2142 = call <vilib>:"Get System Directory.vi"("system directory type"=w5287) -> ("system directory"=w5297:path)  [unwired: 10 in]
                n2143 = Decimate 1D Array(w5318) -> (w5313:dbl[], w5317:dbl[], w5316:dbl[])
                n2144 = for {
                  tunnel: [w5346] -> w5314 mode=indexing
                  tunnel: w5315 -> [w5340] mode=indexing
                  tunnel: w5313 -> [w5339] mode=indexing
                  tunnel: w5317 -> [w5338] mode=indexing
                  tunnel: w5316 -> [w5337] mode=indexing
                  tunnel: [w5339] -> w5312 mode=indexing
                  tunnel: [w5338] -> w5311 mode=indexing
                  tunnel: [w5337] -> w5310 mode=indexing
                  tunnel: w5309 -> [w5332]
                  tunnel: w5308 -> [w5331]
                  tunnel: w5307 -> [w5330] mode=indexing
                  tunnel: w5306 -> [w5329]
                  tunnel: [w5323] -> w5305
                  n2145 = Join Numbers(hi=w5332, lo=w5331) -> ((hi.lo)=w5334:u32)
                  n2146 = To Double Precision Float(number=w5330) -> (double precision float=w5335:dbl)
                  n2147 = Number To Decimal String(number=w5340) -> (decimal integer string=w5345:string)  [unwired: 1 in]
                  n2148 = Number To Fractional String(number=w5339, precision (6)=i16 3 ("width (-)")) -> (F-format string=w5347:string)  [unwired: 2 in]
                  n2149 = Number To Fractional String(number=w5338, precision (6)=i16 3 ("width (-)")) -> (F-format string=w5343:string)  [unwired: 2 in]
                  n2150 = Number To Fractional String(number=w5337, precision (6)=i16 3 ("width (-)")) -> (F-format string=w5341:string)  [unwired: 2 in]
                  n2151 = Build Array(w5345, w5347, w5343, w5341) -> (w5346:string[])
                  n2152 = Divide(x=w5335, y=w5329) -> (x/y=w5336:dbl)
                  n2153 = To Unsigned Quad Integer(1:w5334) -> (0:w5333:u64)
                  n2154 = call "Unix Time to Timestamp.vi"("Fractional Second"=w5336, "Unix Time (s)"=w5333) -> ("Timestamp"=w5324:timestamp)  [unwired: 8 in, 1 out]
                  n2155 = Format Date/Time String(seconds (now)=w5324, UTC format=TRUE) -> (date/time string=w5328:string)  [unwired: 1 in]
                  n2156 = Scan From String(format string="%<%x %H:%M:%S%3u>T", input string=w5328) -> (output 1=w5327:timestamp)  [unwired: 3 in, 3 out]
                  n2157 = To Double Precision Float(number=w5327) -> (double precision float=w5323:dbl)
                }
                n2158 = Build Path(base path=w5297, name or relative path="Logfile") -> (appended path=w5298:path)
                n2159 = call <vilib>:"Check if File or Folder Exists.vi"("path"=w5298) -> ("file or folder exists?"=w5299:bool, "dup path"=w5300:path)  [unwired: 8 in, 1 out]
                n2160 = case shown="False" w5299 {
                  tunnel: w5300 -> [w5321 w5322]
                  tunnel: [w5320 w5322] -> w5301
                  frame False {
                    n2161 = Create Folder(path (use dialog)=w5321) -> (created path=w5320:path)  [unwired: 2 in, 2 out]
                  }
                  frame True {
                  }
                }
                n2162 = Build Path(base path=w5301, name or relative path=w5304) -> (appended path=w5302:path)
                n2163 = Open/Create/Replace File(file path (use dialog)=w5302, operation (0:open)=T11."open or create") -> (refnum out=w5295:refnum<file>, error out=w5293:errorcluster)  [unwired: 4 in, 1 out]
                n2164 = Write to Text File(file (use dialog)=w5295, text=w5296, error in=w5293) -> (refnum out=w5294:refnum<file>, error out=w5292:errorcluster)  [unwired: 1 in, 1 out]
                n2165 = Close File(refnum=w5294, error in=w5292) -> (path=w5281:path)  [unwired: 1 out]
              }
              frame 27 {
                w5356 = T14 2 items=["User Home"=0, "User Desktop"=1, "User Documents"=2, "User Application Data"=3, "User Preferences"=4, "User Temporary"=5, "Public Documents"=6, "Public Application Data"=7, "Public Preferences"=8, "Public Cache"=13, "System Core Libraries"=9, "System Installed Libraries"=10, "Application Files"=11, "Boot Volume Root"=12] ("system directory type")
                n2166 = Search and Replace String(replace all?=TRUE ("replace all? (F)"), input string=w5351, search string="/") -> (result string=w5372:string)  [unwired: 5 in, 3 out]
                n2167 = Concatenate Strings(w5349, "TimeStamp;Measure Ch_Z(g);Ch_X(g);INC_X(Deg);INC_Y(Deg)", "\n") -> (w5365:string)
                n2168 = Concatenate Strings(w5372, "_" ("string"), "S_E_T.csv") -> (w5373:string)
                n2169 = call <vilib>:"Get System Directory.vi"("system directory type"=w5356) -> ("system directory"=w5366:path)  [unwired: 10 in]
                n2170 = Decimate 1D Array(w5389) -> (w5387:dbl[], w5386:dbl[], w5384:dbl[], w5383:dbl[])
                n2171 = for {
                  tunnel: [w5420] -> w5388 mode=indexing
                  tunnel: w5385 -> [w5414] mode=indexing
                  tunnel: w5387 -> [w5411] mode=indexing
                  tunnel: w5386 -> [w5410] mode=indexing
                  tunnel: w5384 -> [w5409] mode=indexing
                  tunnel: w5383 -> [w5408] mode=indexing
                  tunnel: [w5411] -> w5382 mode=indexing
                  tunnel: [w5410] -> w5381 mode=indexing
                  tunnel: [w5409] -> w5380 mode=indexing
                  tunnel: [w5408] -> w5379 mode=indexing
                  tunnel: w5378 -> [w5403]
                  tunnel: w5377 -> [w5402]
                  tunnel: w5376 -> [w5401] mode=indexing
                  tunnel: w5375 -> [w5400]
                  tunnel: [w5394] -> w5374
                  n2172 = Join Numbers(hi=w5403, lo=w5402) -> ((hi.lo)=w5405:u32)
                  n2173 = To Double Precision Float(number=w5401) -> (double precision float=w5406:dbl)
                  n2174 = Number To Decimal String(number=w5414) -> (decimal integer string=w5419:string)  [unwired: 1 in]
                  n2175 = Number To Fractional String(number=w5411, precision (6)=i16 3 ("width (-)")) -> (F-format string=w5421:string)  [unwired: 2 in]
                  n2176 = Number To Fractional String(number=w5410, precision (6)=i16 3 ("width (-)")) -> (F-format string=w5417:string)  [unwired: 2 in]
                  n2177 = Number To Fractional String(number=w5409, precision (6)=i16 3 ("width (-)")) -> (F-format string=w5415:string)  [unwired: 2 in]
                  n2178 = Number To Fractional String(number=w5408, precision (6)=i16 3 ("width (-)")) -> (F-format string=w5412:string)  [unwired: 2 in]
                  n2179 = Build Array(w5419, w5421, w5417, w5415, w5412) -> (w5420:string[])
                  n2180 = Divide(x=w5406, y=w5400) -> (x/y=w5407:dbl)
                  n2181 = To Unsigned Quad Integer(1:w5405) -> (0:w5404:u64)
                  n2182 = call "Unix Time to Timestamp.vi"("Fractional Second"=w5407, "Unix Time (s)"=w5404) -> ("Timestamp"=w5395:timestamp)  [unwired: 8 in, 1 out]
                  n2183 = Format Date/Time String(seconds (now)=w5395, UTC format=TRUE) -> (date/time string=w5396:string)  [unwired: 1 in]
                  n2184 = Scan From String(format string="%<%x %H:%M:%S%3u>T", input string=w5396) -> (output 1=w5397:timestamp)  [unwired: 3 in, 3 out]
                  n2185 = To Double Precision Float(number=w5397) -> (double precision float=w5394:dbl)
                }
                n2186 = Build Path(base path=w5366, name or relative path="Logfile") -> (appended path=w5367:path)
                n2187 = call <vilib>:"Check if File or Folder Exists.vi"("path"=w5367) -> ("file or folder exists?"=w5368:bool, "dup path"=w5369:path)  [unwired: 8 in, 1 out]
                n2188 = case shown="False" w5368 {
                  tunnel: w5369 -> [w5392 w5393]
                  tunnel: [w5391 w5393] -> w5370
                  frame False {
                    n2189 = Create Folder(path (use dialog)=w5392) -> (created path=w5391:path)  [unwired: 2 in, 2 out]
                  }
                  frame True {
                  }
                }
                n2190 = Build Path(base path=w5370, name or relative path=w5373) -> (appended path=w5371:path)
                n2191 = Open/Create/Replace File(file path (use dialog)=w5371, operation (0:open)=T11."open or create") -> (refnum out=w5364:refnum<file>, error out=w5362:errorcluster)  [unwired: 4 in, 1 out]
                n2192 = Write to Text File(file (use dialog)=w5364, text=w5365, error in=w5362) -> (refnum out=w5363:refnum<file>, error out=w5361:errorcluster)  [unwired: 1 in, 1 out]
                n2193 = Close File(refnum=w5363, error in=w5361) -> (path=w5350:path)  [unwired: 1 out]
              }
              frame 28 {
                w5430 = T14 2 items=["User Home"=0, "User Desktop"=1, "User Documents"=2, "User Application Data"=3, "User Preferences"=4, "User Temporary"=5, "Public Documents"=6, "Public Application Data"=7, "Public Preferences"=8, "Public Cache"=13, "System Core Libraries"=9, "System Installed Libraries"=10, "Application Files"=11, "Boot Volume Root"=12] ("system directory type")
                n2194 = Search and Replace String(replace all?=TRUE ("replace all? (F)"), input string=w5425, search string="/") -> (result string=w5446:string)  [unwired: 5 in, 3 out]
                n2195 = Concatenate Strings(w5423, "TimeStamp;Measure Ch_Y(g);INC_X(Deg);INC_Y(Deg)", "\n") -> (w5439:string)
                n2196 = Concatenate Strings(w5446, "_" ("string"), "S_E_T.csv") -> (w5447:string)
                n2197 = call <vilib>:"Get System Directory.vi"("system directory type"=w5430) -> ("system directory"=w5440:path)  [unwired: 10 in]
                n2198 = Decimate 1D Array(w5461) -> (w5459:dbl[], w5458:dbl[], w5457:dbl[])
                n2199 = for {
                  tunnel: [w5489] -> w5456 mode=indexing
                  tunnel: w5460 -> [w5483] mode=indexing
                  tunnel: w5459 -> [w5482] mode=indexing
                  tunnel: w5458 -> [w5481] mode=indexing
                  tunnel: w5457 -> [w5480] mode=indexing
                  tunnel: [w5482] -> w5455 mode=indexing
                  tunnel: [w5481] -> w5454 mode=indexing
                  tunnel: [w5480] -> w5453 mode=indexing
                  tunnel: w5452 -> [w5475]
                  tunnel: w5451 -> [w5474]
                  tunnel: w5450 -> [w5473] mode=indexing
                  tunnel: w5449 -> [w5472]
                  tunnel: [w5466] -> w5448
                  n2200 = Join Numbers(hi=w5475, lo=w5474) -> ((hi.lo)=w5477:u32)
                  n2201 = To Double Precision Float(number=w5473) -> (double precision float=w5478:dbl)
                  n2202 = Number To Decimal String(number=w5483) -> (decimal integer string=w5488:string)  [unwired: 1 in]
                  n2203 = Number To Fractional String(number=w5482, precision (6)=i16 3 ("width (-)")) -> (F-format string=w5490:string)  [unwired: 2 in]
                  n2204 = Number To Fractional String(number=w5481, precision (6)=i16 3 ("width (-)")) -> (F-format string=w5486:string)  [unwired: 2 in]
                  n2205 = Number To Fractional String(number=w5480, precision (6)=i16 3 ("width (-)")) -> (F-format string=w5484:string)  [unwired: 2 in]
                  n2206 = Build Array(w5488, w5490, w5486, w5484) -> (w5489:string[])
                  n2207 = Divide(x=w5478, y=w5472) -> (x/y=w5479:dbl)
                  n2208 = To Unsigned Quad Integer(1:w5477) -> (0:w5476:u64)
                  n2209 = call "Unix Time to Timestamp.vi"("Fractional Second"=w5479, "Unix Time (s)"=w5476) -> ("Timestamp"=w5467:timestamp)  [unwired: 8 in, 1 out]
                  n2210 = Format Date/Time String(seconds (now)=w5467, UTC format=TRUE) -> (date/time string=w5468:string)  [unwired: 1 in]
                  n2211 = Scan From String(format string="%<%x %H:%M:%S%3u>T", input string=w5468) -> (output 1=w5469:timestamp)  [unwired: 3 in, 3 out]
                  n2212 = To Double Precision Float(number=w5469) -> (double precision float=w5466:dbl)
                }
                n2213 = Build Path(base path=w5440, name or relative path="Logfile") -> (appended path=w5441:path)
                n2214 = call <vilib>:"Check if File or Folder Exists.vi"("path"=w5441) -> ("file or folder exists?"=w5442:bool, "dup path"=w5443:path)  [unwired: 8 in, 1 out]
                n2215 = case shown="False" w5442 {
                  tunnel: w5443 -> [w5464 w5465]
                  tunnel: [w5463 w5465] -> w5444
                  frame False {
                    n2216 = Create Folder(path (use dialog)=w5464) -> (created path=w5463:path)  [unwired: 2 in, 2 out]
                  }
                  frame True {
                  }
                }
                n2217 = Build Path(base path=w5444, name or relative path=w5447) -> (appended path=w5445:path)
                n2218 = Open/Create/Replace File(file path (use dialog)=w5445, operation (0:open)=T11."open or create") -> (refnum out=w5438:refnum<file>, error out=w5436:errorcluster)  [unwired: 4 in, 1 out]
                n2219 = Write to Text File(file (use dialog)=w5438, text=w5439, error in=w5436) -> (refnum out=w5437:refnum<file>, error out=w5435:errorcluster)  [unwired: 1 in, 1 out]
                n2220 = Close File(refnum=w5437, error in=w5435) -> (path=w5424:path)  [unwired: 1 out]
              }
              frame 29 {
                w5499 = T14 2 items=["User Home"=0, "User Desktop"=1, "User Documents"=2, "User Application Data"=3, "User Preferences"=4, "User Temporary"=5, "Public Documents"=6, "Public Application Data"=7, "Public Preferences"=8, "Public Cache"=13, "System Core Libraries"=9, "System Installed Libraries"=10, "Application Files"=11, "Boot Volume Root"=12] ("system directory type")
                n2221 = Search and Replace String(replace all?=TRUE ("replace all? (F)"), input string=w5494, search string="/") -> (result string=w5515:string)  [unwired: 5 in, 3 out]
                n2222 = Concatenate Strings(w5492, "TimeStamp;Measure Ch_Z(g);Ch_Y(g);INC_X(Deg);INC_Y(Deg)", "\n") -> (w5508:string)
                n2223 = Concatenate Strings(w5515, "_" ("string"), "S_E_T.csv") -> (w5516:string)
                n2224 = call <vilib>:"Get System Directory.vi"("system directory type"=w5499) -> ("system directory"=w5509:path)  [unwired: 10 in]
                n2225 = Decimate 1D Array(w5532) -> (w5526:dbl[], w5530:dbl[], w5527:dbl[], w5528:dbl[])
                n2226 = for {
                  tunnel: [w5563] -> w5529 mode=indexing
                  tunnel: w5531 -> [w5557] mode=indexing
                  tunnel: w5526 -> [w5554] mode=indexing
                  tunnel: w5530 -> [w5553] mode=indexing
                  tunnel: w5527 -> [w5552] mode=indexing
                  tunnel: w5528 -> [w5551] mode=indexing
                  tunnel: [w5554] -> w5525 mode=indexing
                  tunnel: [w5553] -> w5524 mode=indexing
                  tunnel: [w5552] -> w5523 mode=indexing
                  tunnel: [w5551] -> w5522 mode=indexing
                  tunnel: w5521 -> [w5546]
                  tunnel: w5520 -> [w5545]
                  tunnel: w5519 -> [w5544] mode=indexing
                  tunnel: w5518 -> [w5543]
                  tunnel: [w5537] -> w5517
                  n2227 = Join Numbers(hi=w5546, lo=w5545) -> ((hi.lo)=w5548:u32)
                  n2228 = To Double Precision Float(number=w5544) -> (double precision float=w5549:dbl)
                  n2229 = Number To Decimal String(number=w5557) -> (decimal integer string=w5562:string)  [unwired: 1 in]
                  n2230 = Number To Fractional String(number=w5554, precision (6)=i16 3 ("width (-)")) -> (F-format string=w5564:string)  [unwired: 2 in]
                  n2231 = Number To Fractional String(number=w5553, precision (6)=i16 3 ("width (-)")) -> (F-format string=w5560:string)  [unwired: 2 in]
                  n2232 = Number To Fractional String(number=w5552, precision (6)=i16 3 ("width (-)")) -> (F-format string=w5558:string)  [unwired: 2 in]
                  n2233 = Number To Fractional String(number=w5551, precision (6)=i16 3 ("width (-)")) -> (F-format string=w5555:string)  [unwired: 2 in]
                  n2234 = Build Array(w5562, w5564, w5560, w5558, w5555) -> (w5563:string[])
                  n2235 = Divide(x=w5549, y=w5543) -> (x/y=w5550:dbl)
                  n2236 = To Unsigned Quad Integer(1:w5548) -> (0:w5547:u64)
                  n2237 = call "Unix Time to Timestamp.vi"("Fractional Second"=w5550, "Unix Time (s)"=w5547) -> ("Timestamp"=w5538:timestamp)  [unwired: 8 in, 1 out]
                  n2238 = Format Date/Time String(seconds (now)=w5538, UTC format=TRUE) -> (date/time string=w5539:string)  [unwired: 1 in]
                  n2239 = Scan From String(format string="%<%x %H:%M:%S%3u>T", input string=w5539) -> (output 1=w5540:timestamp)  [unwired: 3 in, 3 out]
                  n2240 = To Double Precision Float(number=w5540) -> (double precision float=w5537:dbl)
                }
                n2241 = Build Path(base path=w5509, name or relative path="Logfile") -> (appended path=w5510:path)
                n2242 = call <vilib>:"Check if File or Folder Exists.vi"("path"=w5510) -> ("file or folder exists?"=w5511:bool, "dup path"=w5512:path)  [unwired: 8 in, 1 out]
                n2243 = case shown="False" w5511 {
                  tunnel: w5512 -> [w5535 w5536]
                  tunnel: [w5534 w5536] -> w5513
                  frame False {
                    n2244 = Create Folder(path (use dialog)=w5535) -> (created path=w5534:path)  [unwired: 2 in, 2 out]
                  }
                  frame True {
                  }
                }
                n2245 = Build Path(base path=w5513, name or relative path=w5516) -> (appended path=w5514:path)
                n2246 = Open/Create/Replace File(file path (use dialog)=w5514, operation (0:open)=T11."open or create") -> (refnum out=w5507:refnum<file>, error out=w5505:errorcluster)  [unwired: 4 in, 1 out]
                n2247 = Write to Text File(file (use dialog)=w5507, text=w5508, error in=w5505) -> (refnum out=w5506:refnum<file>, error out=w5504:errorcluster)  [unwired: 1 in, 1 out]
                n2248 = Close File(refnum=w5506, error in=w5504) -> (path=w5493:path)  [unwired: 1 out]
              }
              frame 30 {
